vi "GetTemperatureImage(SubVI).vi"(0 "Refnum in":refnum<k35>, 1 "Temperature Range (High)":dbl, 2 "Temperature Range (Low)":dbl) -> (7 "Temperature array out":dbl[][](array[numeric]))   [LabVIEW 2020]
panel:
  in  "Array Type in":dbl[](array[numeric])
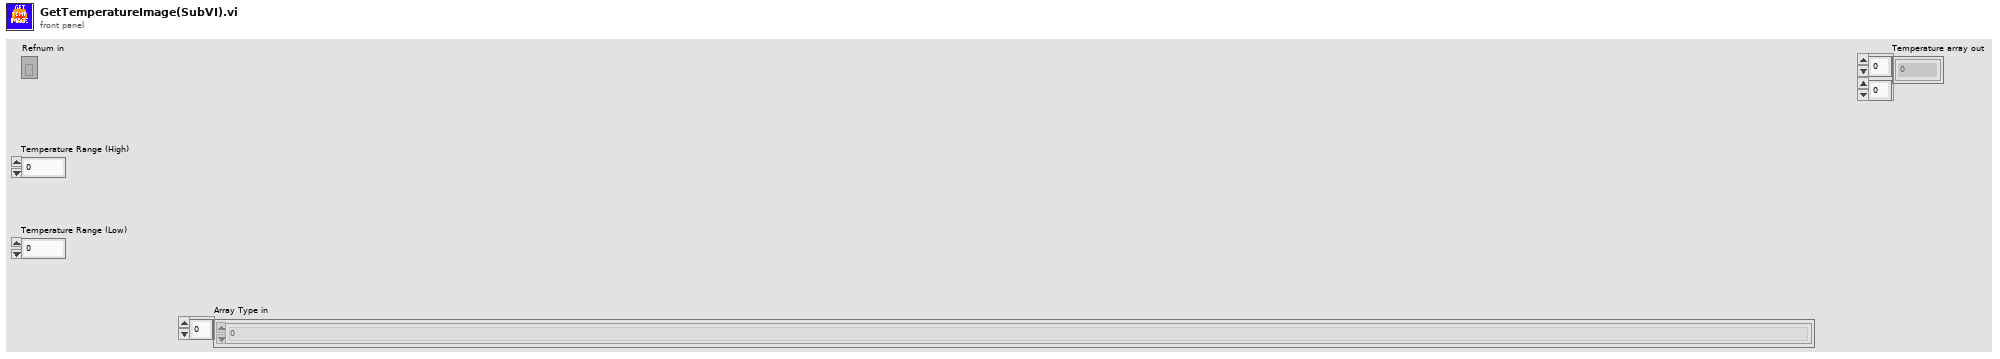
[diagram p1: front panel]
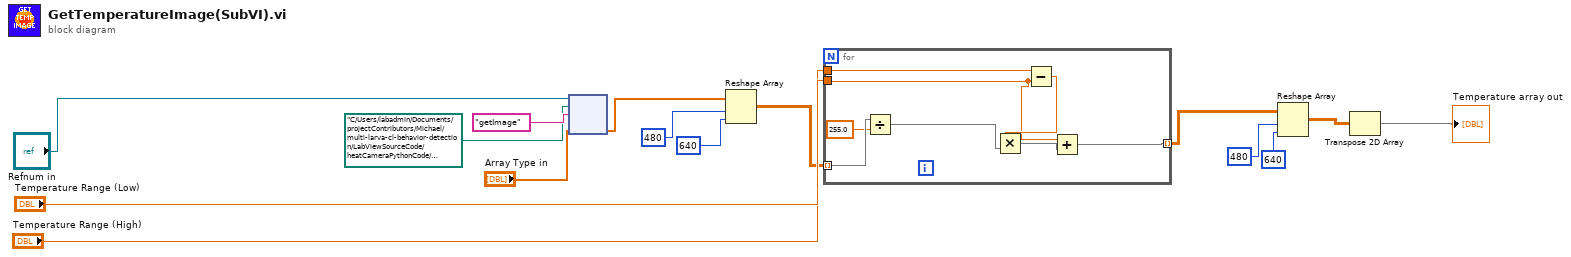
[diagram p0: block diagram]
diagram:
  n1 = node("Refnum in", path "C:/Users/labadmin/Documents/projectContributors/Michael/multi-larva-cl-behavior-detection/LabViewSourceCode/heatCameraPythonCode/customFlir.py" ("module path"), "getImage" ("function name"), "Array Type in") -> (w12:dbl[])  [unwired: 1 in, 4 out]
  n2 = Reshape Array(w12, 480 ("dimension size"), 640 ("dimension size")) -> (w1:dbl[][])
  n3 = for {
    tunnel: w1 -> [w23] mode=indexing
    tunnel: [w18] -> w4 mode=indexing
    tunnel: "Temperature Range (High)" -> [w17]
    tunnel: "Temperature Range (Low)" -> [w16]
    n4 = Divide(x=w23, y=255.0) -> (x/y=w21:dbl[])
    n5 = Subtract(x=w17, y=w16) -> (x-y=w20:dbl)
    n6 = Multiply(x=w20, y=w21) -> (x*y=w19:dbl[])
    n7 = Add(x=w16, y=w19) -> (x+y=w18:dbl[])
  }
  n8 = Reshape Array(w4, 480 ("dimension size"), 640 ("dimension size")) -> (w5:dbl[][])
  n9 = Transpose 2D Array(2D array=w5) -> (transposed array=→"Temperature array out":dbl[][])
